vi "Calculate Byte Start Address.vi"(9 "data_byte_alignment":i32=1, 10 "byte_address_start":i32) -> (2 "bytes_padding":i32, 3 "byte_address_data":i32)   [LabVIEW 2021, in "DataTypes_CIF_U.lvlib"]
uses:
  DataTypes_CIF_U.lvlib
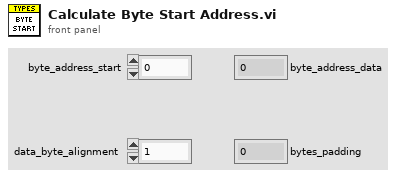
[diagram p1: front panel]
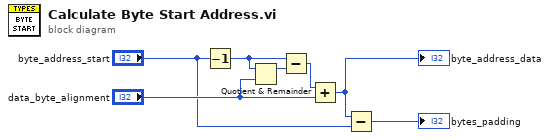
[diagram p0: block diagram]
diagram:
  n1 = Decrement(x="byte_address_start") -> (x-1=w1:i32)
  n2 = Quotient & Remainder(x=w1, y="data_byte_alignment") -> (x-y*floor(x/y)=w3:i32)  [unwired: 1 out]
  n3 = Subtract(x=w1, y=w3) -> (x-y=w2:i32)
  n4 = Add(x=w2, y="data_byte_alignment") -> (x+y=w6:i32)
  "byte_address_data" <- w6
  n5 = Subtract(x=w6, y="byte_address_start") -> (x-y=→"bytes_padding":i32)
